vi "EE_CreateXMLHeader.vi"(2 "UserName":string) -> (0 "XML_Header out":T2)   [LabVIEW 2016, in "Emotiv Epoc.lvlib"]
uses:
  Emotiv Epoc.lvlib
  _XML_EEG_File_Parser/_vlib/XML_EEG_Header.ctl
  Emotiv_EEG_Channels_enum.ctl
  _XML_EEG_File_Parser/XML_EEG_File_Parser.lvlib
panel:
  in  "Emotiv_EEG_Channels_enum":T1
  # "This VI is a part of BCI Design library, http://www.ru-bci.org \nCopyright © 2020, Sotnikov Peter, All rights reserved. License: GNU GPLv3"
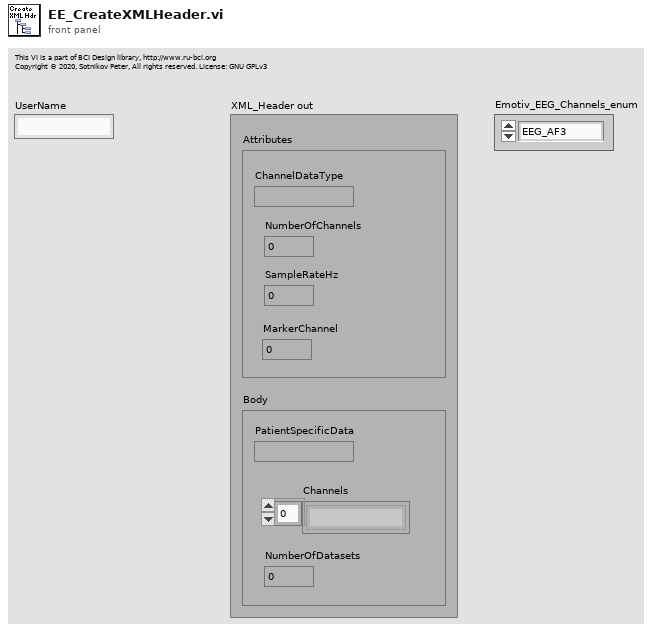
[diagram p1: front panel]
types:
  T1 = typedef "Emotiv Epoc.lvlib/Emotiv_EEG_Channels_enum.ctl" = enum16{"EEG_AF3", "EEG_F7", "EEG_F3", "EEG_FC5", "EEG_T7", "EEG_P7", "EEG_O1", "EEG_O2", "EEG_P8", "EEG_T8", "EEG_FC6", "EEG_F4", "EEG_F8", "EEG_AF4"}
  T2 = typedef "XML_EEG_File_Parser.lvlib/XML_EEG_Header.ctl" = cluster{"Attributes":cluster{"ChannelDataType":string, "NumberOfChannels":i32, "SampleRateHz":dbl, "MarkerChannel":i32}, "Body":cluster{"PatientSpecificData":string, "NumberOfDatasets":i32, "Channels":string[]}}
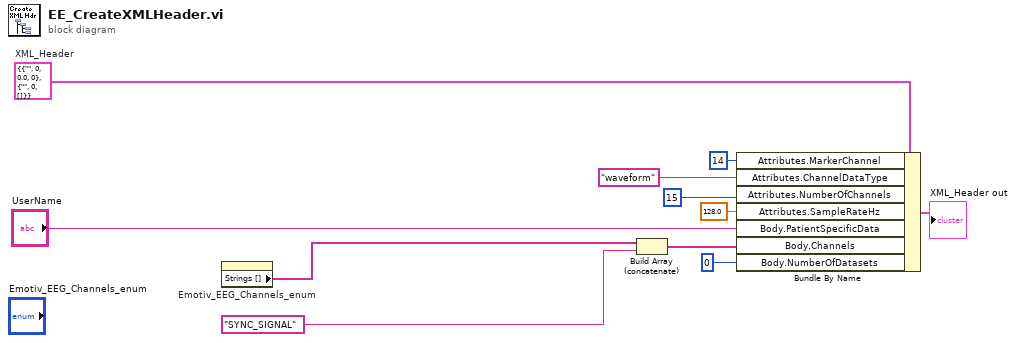
[diagram p0: block diagram]
diagram:
  w11 = T2 {"Attributes"={"ChannelDataType"="", "NumberOfChannels"=0, "SampleRateHz"=0.0, "MarkerChannel"=0}, "Body"={"PatientSpecificData"="", "NumberOfDatasets"=0, "Channels"=[]}}  # XML_Header
  n1 = property on="Emotiv_EEG_Channels_enum" class="Enum (strict)"() -> ("Strings []"=w3:string[])  [unwired: 2 in, 2 out]
  n2 = Build Array (concatenate)(w3, "SYNC_SIGNAL") -> (w2:string[])
  n3 = Bundle By Name(cluster=w11, "Attributes.MarkerChannel"=14, "Attributes.ChannelDataType"="waveform", "Attributes.NumberOfChannels"=15, "Attributes.SampleRateHz"=128.0, "Body.PatientSpecificData"="UserName", "Body.Channels"=w2, "Body.NumberOfDatasets"=0) -> (→"XML_Header out":T2)
